vi "Pre Launch Init.vi"(11 "SW_Interface_Class in":refnum<class "SW_Interface_Class.lvclass">) -> (0 "error out":errorcluster, 3 "SW_Interface_Class out":refnum<class "SW_Interface_Class.lvclass">)   [LabVIEW 2023, in "SW_Interface_Actor.lvlib" / "SW_Interface_Class.lvclass"]
doc: "(<B>Filename</B>: Actor Framework.lvlib:Actor.lvclass:Pre Launch Init.vi)\n\nDefines behavior that occurs after the Launch Nested Actor method is invoked but before the actor's Actor Core method begins running.\n\nBy default, this method does nothing. A descendant class may override it to define behavior."
uses:
  SW_Interface_Class.lvclass
  Abstraction_Interface_Class/Abstraction_Interface_Class.lvclass
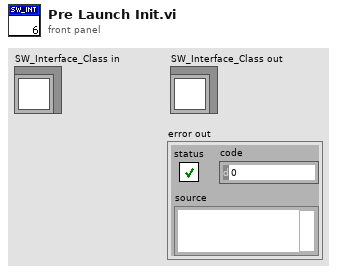
[diagram p1: front panel]
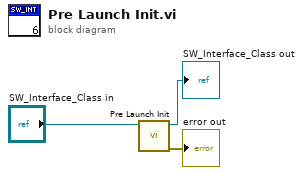
[diagram p0: block diagram]
diagram:
  n1 = call-parent "Pre Launch Init.vi"("Actor in"="SW_Interface_Class in") -> ("error out"=→"error out":errorcluster, "Actor out"=→"SW_Interface_Class out":refnum<class "SW_Interface_Class.lvclass">)  [unwired: 9 in]
